vi "排气扇监测界面.vi"() -> ()   [LabVIEW 2016, in "环境动力监测库.lvlib"]
uses:
  <vilib>/Utility/config.llb/NI_LVConfig.lvlib
  <vilib>/ptbypt/NI_PtbyPt.lvlib
panel:
  in  "功能开关":enum16{"关闭", "开启"}(ring)
  in  "排气扇关闭温度":dbl=60.0 caption="关闭温度" format="%#_2f ℃"
  in  "排气扇开启温度":dbl=60.0 caption="开启温度" format="%#.2f ℃"
  in  "排气扇":bool
  # "排气扇监测"
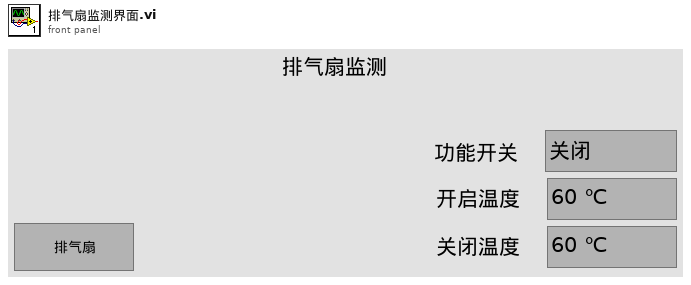
[diagram p1: front panel]
types:
  T1 = cluster{"功能开关":enum16{"关闭", "开启"}, "排气扇开启温度":dbl, "排气扇关闭温度":dbl}
  T2 = cluster{"漏水监测配置":cluster{"监测项描述:输出":string, "端口:":enum16{"AI0", "AI1", "AI2", "AI3", "AI4", "DI0", "DI1", "DI2", "DI3", "DI4", "DO0", "DO1", "DO2", "DO3", "DO4", "X0", "X1", "X2", "X3", "X4", "X5", "X6", "X7", "X8", "X9"}, "告警参数:":enum32{"禁用告警", "闭合告警", "断开告警"}, "传感器型号:":enum16{"PLC", "ZLAN"}}, "门禁开关监测配置":cluster{"监测项描述:输出":string, "端口:":enum16{"AI0", "AI1", "AI2", "AI3", "AI4", "DI0", "DI1", "DI2", "DI3", "DI4", "DO0", "DO1", "DO2", "DO3", "DO4", "X0", "X1", "X2", "X3", "X4", "X5", "X6", "X7", "X8", "X9"}, "告警参数:":enum32{"禁用告警", "闭合告警", "断开告警"}, "传感器型号:":enum16{"PLC", "ZLAN"}}, "温湿度监测配置":cluster{"监测项描述:输出":string, "端口:":enum16{"AI0", "AI1", "AI2", "AI3", "AI4", "DI0", "DI1", "DI2", "DI3", "DI4", "DO0", "DO1", "DO2", "DO3", "DO4", "X0", "X1", "X2", "X3", "X4", "X5", "X6", "X7", "X8", "X9"}, "告警参数:":enum32{"禁用告警", "闭合告警", "断开告警"}, "传感器型号:":enum16{"PLC", "ZLAN"}}, "烟雾监测配置":cluster{"监测项描述:输出":string, "端口:":enum16{"AI0", "AI1", "AI2", "AI3", "AI4", "DI0", "DI1", "DI2", "DI3", "DI4", "DO0", "DO1", "DO2", "DO3", "DO4", "X0", "X1", "X2", "X3", "X4", "X5", "X6", "X7", "X8", "X9"}, "告警参数:":enum32{"禁用告警", "闭合告警", "断开告警"}, "传感器型号:":enum16{"PLC", "ZLAN"}}, "冰箱监测配置":cluster{"监测项描述:输出":string, "端口:":enum16{"AI0", "AI1", "AI2", "AI3", "AI4", "DI0", "DI1", "DI2", "DI3", "DI4", "DO0", "DO1", "DO2", "DO3", "DO4", "X0", "X1", "X2", "X3", "X4", "X5", "X6", "X7", "X8", "X9"}, "告警参数:":enum32{"禁用告警", "闭合告警", "断开告警"}, "传感器型号:":enum16{"PLC", "ZLAN"}}, "排气扇监测配置":cluster{"监测项描述:输出":string, "端口:":enum16{"AI0", "AI1", "AI2", "AI3", "AI4", "DI0", "DI1", "DI2", "DI3", "DI4", "DO0", "DO1", "DO2", "DO3", "DO4", "X0", "X1", "X2", "X3", "X4", "X5", "X6", "X7", "X8", "X9"}, "告警参数:":enum32{"禁用告警", "闭合告警", "断开告警"}, "传感器型号:":enum16{"PLC", "ZLAN"}}}
  T3 = cluster{"监测项描述:输出":string, "端口:":enum16{"AI0", "AI1", "AI2", "AI3", "AI4", "DI0", "DI1", "DI2", "DI3", "DI4", "DO0", "DO1", "DO2", "DO3", "DO4", "X0", "X1", "X2", "X3", "X4", "X5", "X6", "X7", "X8", "X9"}, "告警参数:":enum32{"禁用告警", "闭合告警", "断开告警"}, "传感器型号:":enum16{"PLC", "ZLAN"}}
  T4 = enum16{"AI0", "AI1", "AI2", "AI3", "AI4", "DI0", "DI1", "DI2", "DI3", "DI4", "DO0", "DO1", "DO2", "DO3", "DO4", "X0", "X1", "X2", "X3", "X4", "X5", "X6", "X7", "X8", "X9"}
  T5 = cluster{"状态":cluster{"R0":i16, "R1":i16, "R2":i16, "R3":i16, "R4":i16, "R5":i16, "R6":i16, "R7":i16, "R8":i16, "R9":i16, "R10":i16, "R11":i16, "R12":i16, "R13":i16, "R14":i16, "R15":i16, "R16":i16, "R17":i16, "R18":i16, "R19":i16, "R20":i16, "R21":i16, "R22":i16, "R23":i16, "R24":i16, "R25":i16, "R26":i16, "R27":i16, "R28":i16, "R29":i16, "R30":i16, "R31":i16, "R32":i16, "R33":i16, "R34":i16, "R35":i16, "R36":i16, "R37":i16, "R38":i16, "R39":i16}, "输入状态":bool[], "输出状态":bool[], "参数设置":cluster{"R100":i16, "R101":i16, "R102":i16, "R103":i16, "R104":i16, "R105":i16, "R106":i16, "R107":i16, "R108":i16, "R109":i16, "R110":i16, "R111":i16, "R112":i16, "R113":i16, "R114":i16, "R115":i16, "R116":i16, "R117":i16, "R118":i16, "R119":i16, "R120":i16, "R121":i16, "R122":i16, "R123":i16}, "转换值":cluster{"AD0":sgl, "AD1":sgl, "AD2":sgl, "AD3":sgl, "AD4":sgl, "AD5":sgl}}
  T6 = cluster{"环境变量":cluster{"蓄电池电压":dbl, "室温":dbl, "湿度":dbl, "水浸报警":bool, "烟雾报警":bool, "门禁1状态":bool, "门禁2状态":bool}, "ZLAN 6842 MB session":refnum<class "MB_Master.lvclass">, "DI":bool[], "DO":bool[], "AD当前转换值":cluster{"AD0":dbl, "AD1":dbl, "AD2":dbl, "AD3":dbl, "AD4":dbl, "AD5":dbl, "AD6":dbl, "AD7":dbl}}
  T7 = typedef "NI_LVConfig.lvlib/Config Data RefNum.ctl" = refnum<k1>
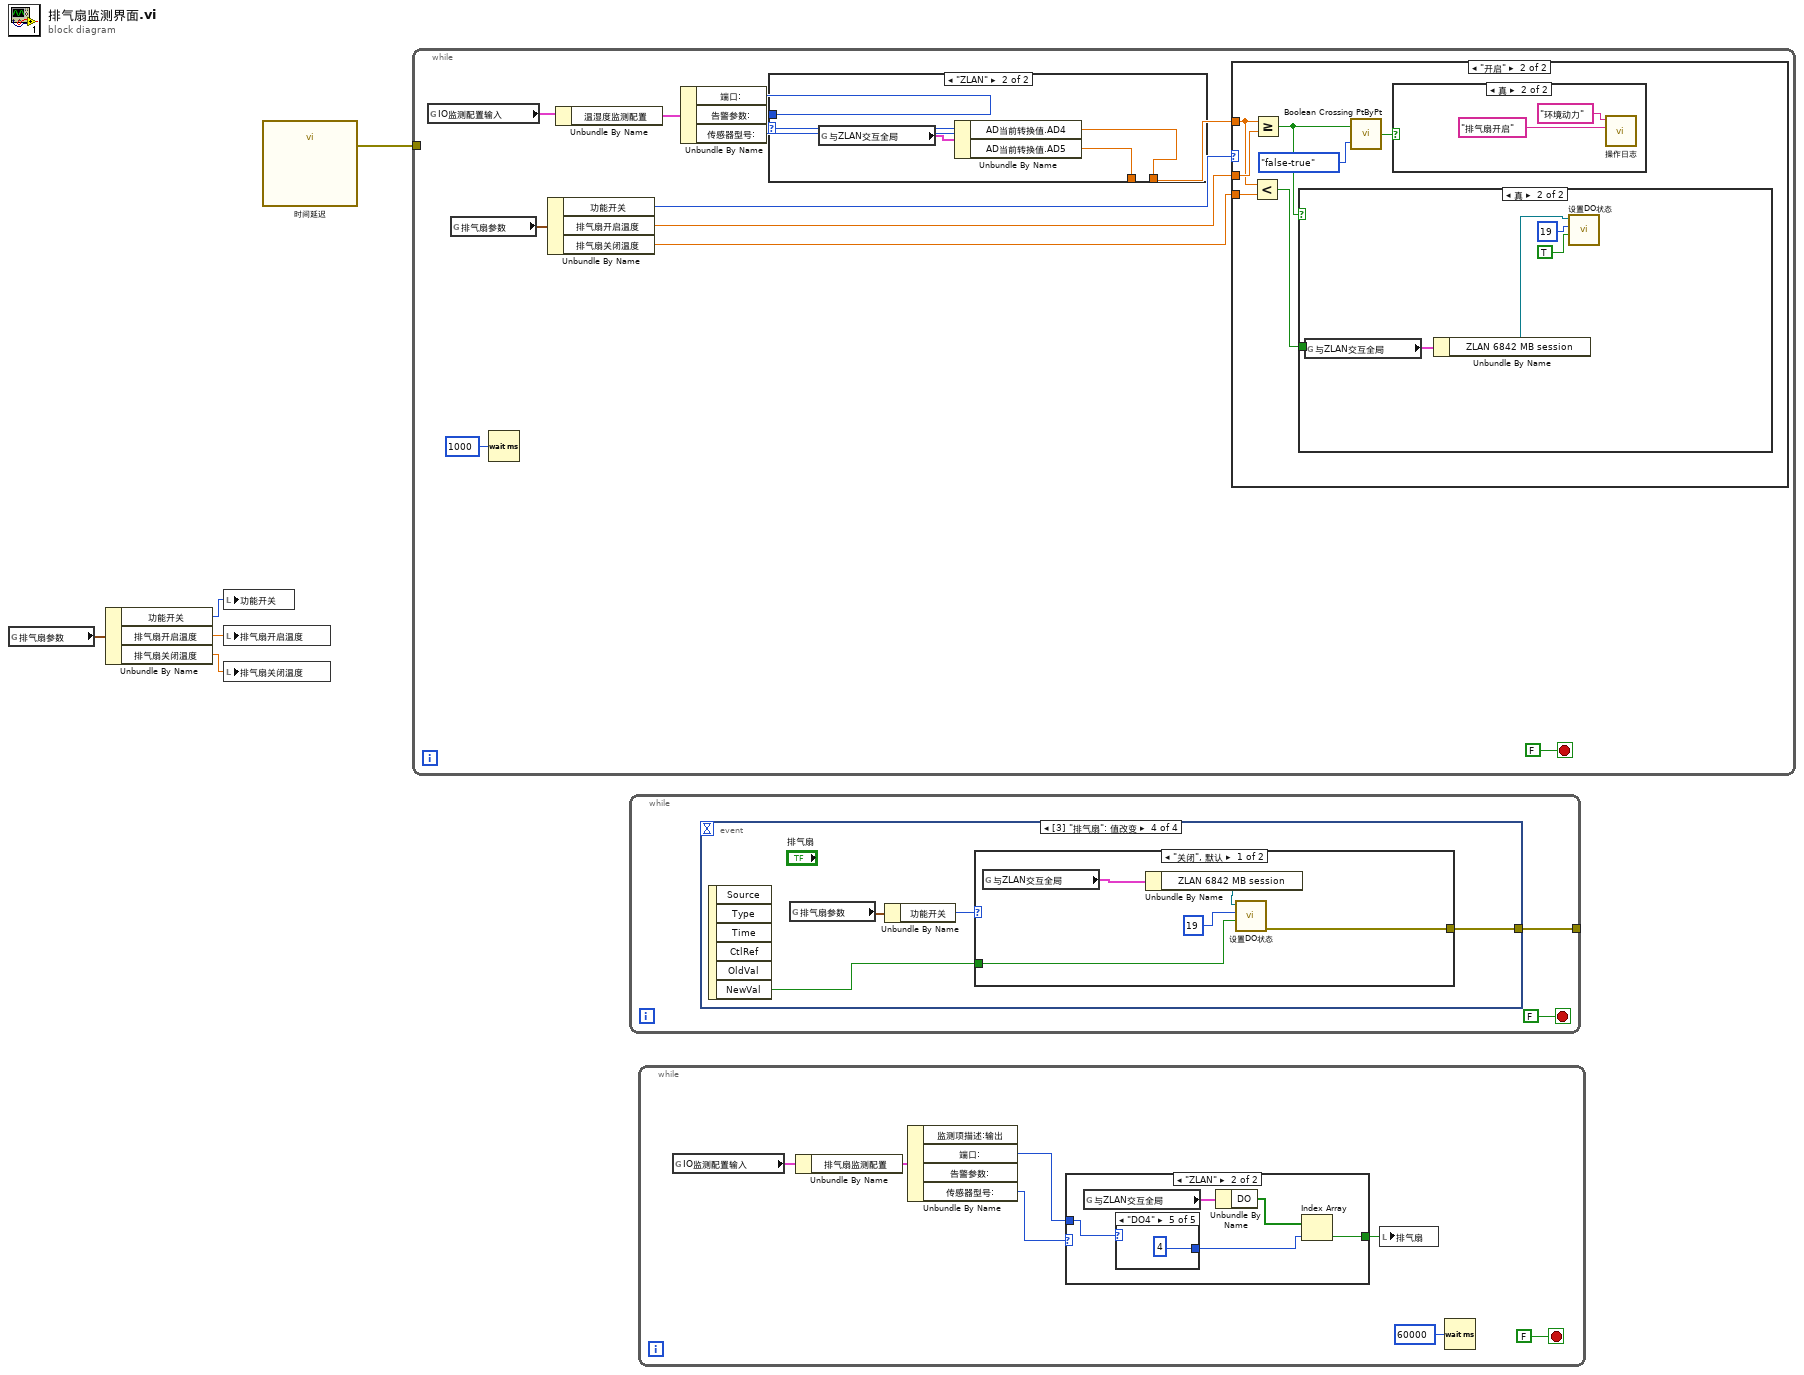
[diagram p0: block diagram]
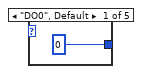
[diagram p3: hidden frame]
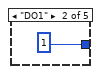
[diagram p4: hidden frame]
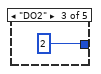
[diagram p5: hidden frame]
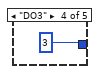
[diagram p6: hidden frame]
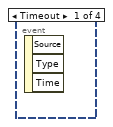
[diagram p7: hidden frame]
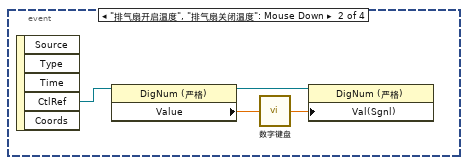
[diagram p8: hidden frame]
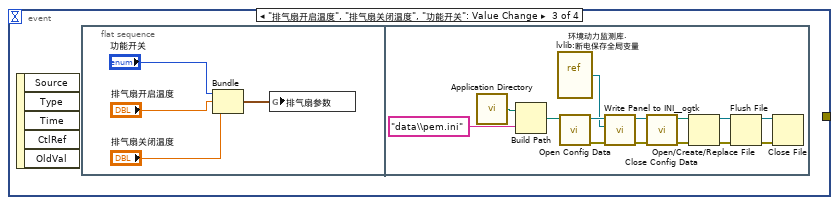
[diagram p9: hidden frame]
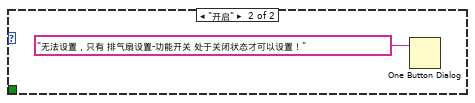
[diagram p10: hidden frame]
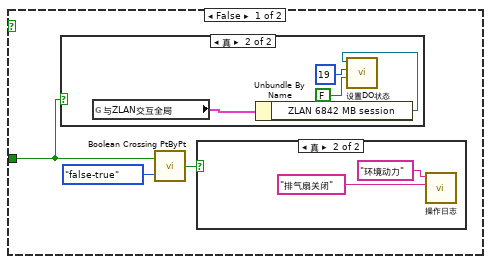
[diagram p13: hidden frame]
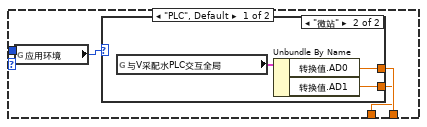
[diagram p16: hidden frame]
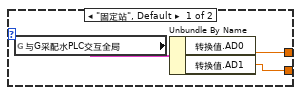
[diagram p17: hidden frame]
diagram:
  n1 = global read "断电保存全局变量.vi" "排气扇参数"() -> (w5:T1)
  n2 = Unbundle By Name(w5) -> ("功能开关"=w4:enum16{"关闭", "开启"}, "排气扇开启温度"=w3:dbl, "排气扇关闭温度"=w2:dbl)
  n3 = local write "功能开关"(w4) -> ()
  n4 = local write "排气扇开启温度"(w3) -> ()
  n5 = local write "排气扇关闭温度"(w2) -> ()
  n6 = call "时间延迟"() -> ("error out"=w1:errorcluster)  [unwired: 11 in]
  n7 = while {
    tunnel: w1 -> [_]
    stop <- FALSE stop-if-true
    n8 = global read "断电保存全局变量.vi" "IO监测配置输入"() -> (w6:T2)
    n9 = global read "断电保存全局变量.vi" "排气扇参数"() -> (w11:T1)
    n10 = Wait (ms)(milliseconds to wait=u32 1000 ("等待时间（毫秒）")) -> ()  [unwired: 1 out]
    n11 = Unbundle By Name(w11) -> ("功能开关"=w9:enum16{"关闭", "开启"}, "排气扇开启温度"=w8:dbl, "排气扇关闭温度"=w7:dbl)
    n12 = Unbundle By Name(w6) -> ("温湿度监测配置"=w14:T3)
    n13 = Unbundle By Name(w14) -> ("端口:"=w12:T4, "传感器型号:"=w13:enum16{"PLC", "ZLAN"})  [unwired: 1 out]
    n14 = case shown="\"ZLAN\"" w13 {
      tunnel: w12 -> [_ _]
      tunnel: [w40 w49] -> w10
      tunnel: [w39 w48] -> _
      frame "PLC", Default {
        n15 = global read "外部交互全局变量.vi" "应用环境"() -> (w41:enum16{"固定站", "微站", "浮标", "浮船"})
        n16 = case shown="\"微站\"" w41 {
          tunnel: [w43 w46] -> w40
          tunnel: [w42 w45] -> w39
          frame "固定站", Default {
            n17 = global read "外部交互全局变量.vi" "与G采配水PLC交互全局"() -> (w44:T5)
            n18 = Unbundle By Name(w44) -> ("转换值.AD0"=w43:sgl, "转换值.AD1"=w42:sgl)
          }
          frame "微站" {
            n19 = global read "外部交互全局变量.vi" "与V采配水PLC交互全局"() -> (w47:T5)
            n20 = Unbundle By Name(w47) -> ("转换值.AD0"=w46:sgl, "转换值.AD1"=w45:sgl)
          }
        }
      }
      frame "ZLAN" {
        n21 = global read "外部交互全局变量.vi" "与ZLAN交互全局"() -> (w50:T6)
        n22 = Unbundle By Name(w50) -> ("AD当前转换值.AD4"=w49:dbl, "AD当前转换值.AD5"=w48:dbl)
      }
    }
    n23 = case shown="\"开启\"" w9 {
      tunnel: w8 -> [_ w19]
      tunnel: w7 -> [_ w18]
      tunnel: w10 -> [_ w17]
      frame "关闭", Default {
      }
      frame "开启" {
        n24 = Less?(x=w17, y=w18) -> (x < y?=w23:bool)
        n25 = Greater Or Equal?(x=w17, y=w19) -> (x >= y?=w22:bool)
        n26 = case shown="真" w22 {
          tunnel: w23 -> [w26 _]
          frame False {
            n27 = case shown="真" w26 {
              frame False {
              }
              frame True {
                n28 = global read "外部交互全局变量.vi" "与ZLAN交互全局"() -> (w32:T6)
                n29 = Unbundle By Name(w32) -> ("ZLAN 6842 MB session"=w31:refnum<class "MB_Master.lvclass">)
                n30 = call "设置DO状态.vi"("value"=FALSE, "address"=u16 19, "MB session in"=w31) -> ()  [unwired: 7 in, 2 out]
              }
            }
            n31 = call <vilib>:"Boolean Crossing PtByPt.vi"("direction"=enum16{"either", "false-true", "true-false"}."false-true", "input"=w26) -> ("crossing"=w27:bool)  [unwired: 1 in]
            n32 = case shown="真" w27 {
              frame False {
              }
              frame True {
                n33 = call "操作日志.vi"("日志信息"="排气扇关闭", "设备"="环境动力") -> ()  [unwired: 9 in, 1 out]
              }
            }
          }
          frame True {
            n34 = global read "外部交互全局变量.vi" "与ZLAN交互全局"() -> (w36:T6)
            n35 = Unbundle By Name(w36) -> ("ZLAN 6842 MB session"=w35:refnum<class "MB_Master.lvclass">)
            n36 = call "设置DO状态.vi"("value"=TRUE, "address"=u16 19, "MB session in"=w35) -> ()  [unwired: 7 in, 2 out]
          }
        }
        n37 = call <vilib>:"Boolean Crossing PtByPt.vi"("direction"=enum16{"either", "false-true", "true-false"}."false-true", "input"=w22) -> ("crossing"=w21:bool)  [unwired: 1 in]
        n38 = case shown="真" w21 {
          frame False {
          }
          frame True {
            n39 = call "操作日志.vi"("日志信息"="排气扇开启", "设备"="环境动力") -> ()  [unwired: 9 in, 1 out]
          }
        }
      }
    }
  }
  n40 = while {
    tunnel: [w51] -> _
    stop <- FALSE stop-if-true
    n41 = event shown="[3] \"排气扇\": 值改变" {
      selector: _ -> [_ _ _ _]
      dyn-events: _ -> [_ _ _ _]
      timeout: _ -> [_ _ _ _]
      tunnel: [_ _ _ w75] -> w51
      event Timeout {
        n42 = event-data() -> ()  [unwired: 1 in, 3 out]
      }
      event "排气扇开启温度", "排气扇关闭温度": Mouse Down {
        n43 = event-data() -> ("CtlRef"=w53:refnum<vi>)  [unwired: 1 in, 4 out]
        n44 = property class="DigNum (严格)"(reference=w53) -> (reference out=w54:refnum<vi>, "Value"=w56:dbl)  [unwired: 1 in, 1 out]
        n45 = call "数字键盘.vi"("OldNumber"=w56) -> ("NewNumber"=w55:sgl)
        n46 = property class="DigNum (严格)"(reference=w54, "Val(Sgnl)"=w55) -> ()  [unwired: 1 in, 2 out]
      }
      event "排气扇开启温度", "排气扇关闭温度", "功能开关": Value Change {
        n47 = event-data() -> ()  [unwired: 1 in, 5 out]
        n48 = flat-sequence {
          frame #0 {
            n49 = Bundle("功能开关"="功能开关", "排气扇开启温度"="排气扇开启温度", "排气扇关闭温度"="排气扇关闭温度") -> (w57:T1)  [unwired: 1 in]
            n50 = global write "断电保存全局变量.vi" "排气扇参数"(w57) -> ()
          }
          frame #1 {
            n51 = call <vilib>:"Application Directory.vi"() -> ("Application Directory"=w74:path)
            n52 = Build Path(base path=w74, name or relative path="data\\pem.ini" ("名称或相对路径")) -> (appended path=w72:path)
            n53 = vi-ref "环境动力监测库.lvlib:断电保存全局变量.vi"() -> (w70:refnum<vi>)
            n54 = call <vilib>:"Open Config Data.vi"("configuration file path"=w72) -> ("error out"=w68:errorcluster, "refnum"=w71:T7)  [unwired: 8 in, 1 out]
            n55 = call <userlib>:"Write Panel to INI__ogtk.vi"("error in (no error)"=w68, "VI ref"=w70, "refnum"=w71) -> ("error out"=w67:errorcluster, "refnum out"=w69:T7)  [unwired: 7 in]
            n56 = call <vilib>:"Close Config Data.vi"("error in (no error)"=w67, "refnum"=w69) -> ("error out"=w62:errorcluster, "file path"=w61:path)  [unwired: 8 in]
            n57 = Open/Create/Replace File(file path (use dialog)=w61, error in=w62) -> (refnum out=w65:refnum<file>, error out=w66:errorcluster)  [unwired: 4 in, 1 out]
            n58 = Flush File(refnum=w65, error in=w66) -> (refnum out=w64:refnum<file>, error out=w63:errorcluster)
            n59 = Close File(refnum=w64, error in=w63) -> ()  [unwired: 2 out]
          }
        }
      }
      event "排气扇": Value Change {
        n60 = event-data() -> ("NewVal"=w76:bool)  [unwired: 1 in, 5 out]
        n61 = global read "断电保存全局变量.vi" "排气扇参数"() -> (w78:T1)
        n62 = Unbundle By Name(w78) -> ("功能开关"=w77:enum16{"关闭", "开启"})
        n63 = case shown="\"关闭\", 默认" w77 {
          tunnel: w76 -> [w82 _]
          tunnel: [w81 _] -> w75
          frame "关闭", Default {
            n64 = global read "外部交互全局变量.vi" "与ZLAN交互全局"() -> (w80:T6)
            n65 = Unbundle By Name(w80) -> ("ZLAN 6842 MB session"=w79:refnum<class "MB_Master.lvclass">)
            n66 = call "设置DO状态.vi"("value"=w82, "address"=u16 19, "MB session in"=w79) -> ("error out"=w81:errorcluster)  [unwired: 7 in, 1 out]
          }
          frame "开启" {
            n67 = One Button Dialog(message="无法设置，只有 排气扇设置-功能开关 处于关闭状态才可以设置！" ("消息")) -> ()  [unwired: 1 in, 1 out]
          }
        }
      }
    }
  }
  n68 = while {
    stop <- FALSE stop-if-true
    n69 = global read "断电保存全局变量.vi" "IO监测配置输入"() -> (w85:T2)
    n70 = Unbundle By Name(w85) -> ("排气扇监测配置"=w89:T3)
    n71 = Unbundle By Name(w89) -> ("端口:"=w87:T4, "传感器型号:"=w88:enum16{"PLC", "ZLAN"})  [unwired: 2 out]
    n72 = case shown="\"ZLAN\"" w88 {
      tunnel: w87 -> [_ w96]
      tunnel: [_ w94] -> w86
      frame "PLC", Default {
      }
      frame "ZLAN" {
        n73 = global read "外部交互全局变量.vi" "与ZLAN交互全局"() -> (w93:T6)
        n74 = case shown="\"DO4\"" w96 {
          tunnel: [0 1 2 3 4] -> w95
          frame "DO0", Default {
          }
          frame "DO1" {
          }
          frame "DO2" {
          }
          frame "DO3" {
          }
          frame "DO4" {
          }
        }
        n75 = Unbundle By Name(w93) -> ("DO"=w92:bool[])
        n76 = Index Array(array=w92, index=w95) -> (element=w94:bool)
      }
    }
    n77 = local write "排气扇"(w86) -> ()
    n78 = Wait (ms)(milliseconds to wait=u32 60000 ("等待时间（毫秒）")) -> ()  [unwired: 1 out]
  }
